vi "get Phasor Config.vi"(7 "phasorIndex":i32, 9 "pmuIndex":i32, 10 "pseudoPdcId":i32, 11 "phasorCfg":T1) -> (1 "function return":i32, 2 "name":string, 3 "phasorCfg out":T1)   [LabVIEW 2013, in "C37118-DLL.lvlib" / "StrongridDLL.lvlib"]
doc: "STRONGRIDIEEEC37118DLL_API int __cdecl getPhasorConfig(phasorConfig *phasorCfg, int32_t pseudoPdcId, int32_t pmuIndex, int32_t phasorIndex);"
uses:
  StrongridDLL.lvlib
  <vilib>/Utility/importsl/GetValueByPointer/datatype.ctl
  <vilib>/Utility/importsl/GetValueByPointer/GetValueByPointer.xnode
  StrongridDLL.dll
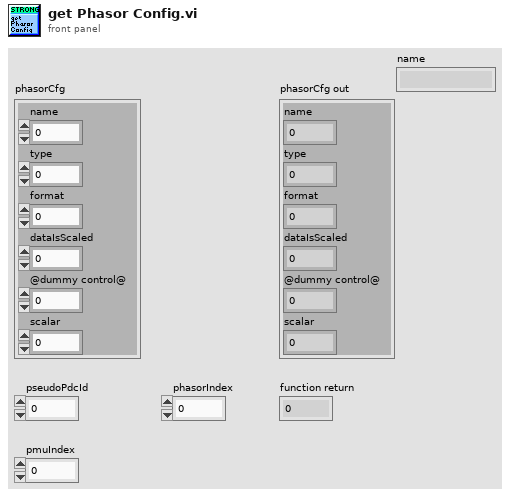
[diagram p1: front panel]
types:
  T1 = cluster{"name":u32, "type":u8, "format":u8, "dataIsScaled":u8, "@dummy control@":i8, "scalar":sgl}
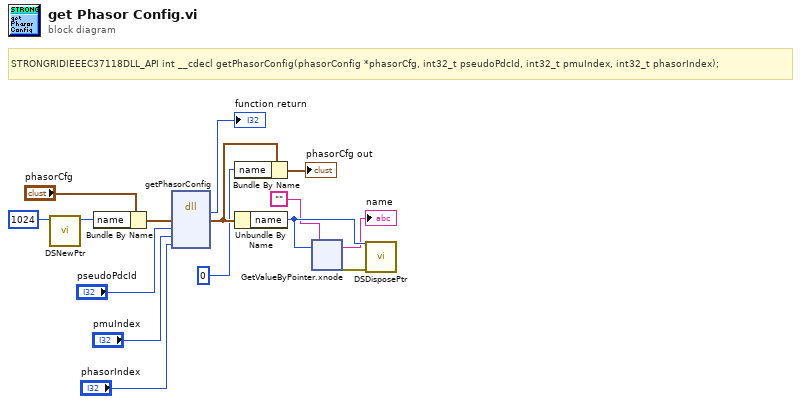
[diagram p0: block diagram]
diagram:
  # "STRONGRIDIEEEC37118DLL_API int __cdecl getPhasorConfig(phasorConfig *phasorCfg, int32_t pseudoPdcId, int32_t pmuIndex, int32_t phasorIndex);"
  n1 = call <vilib>:"DSNewPtr.vi"("Size"=u64 1024) -> ("Pointer"=w12:u64)  [unwired: 9 in, 1 out]
  n2 = Bundle By Name(cluster="phasorCfg", "name"=w12) -> (w11:T1)
  n3 = dll-call lib="C:/dev/statnett/S3DK-Startup/LabVIEW PRL Library LV2013/c37118-dll/labview/vi/Auto Generated/StrongridDLL.*" fn="getPhasorConfig"("phasorCfg"=w11, "pseudoPdcId"="pseudoPdcId", "pmuIndex"="pmuIndex", "phasorIndex"="phasorIndex") -> (→"function return":i32, "phasorCfg"=w6:T1)  [unwired: 6 in, 2 out]
  n4 = Bundle By Name(cluster=w6, "name"=u32 0) -> (→"phasorCfg out":T1)
  n5 = Unbundle By Name(w6) -> ("name"=w9:u32)
  n6 = xnode "GetValueByPointer.xnode"("Pointer"=w9, "InputType"="") -> ("Output"=→"name":string, "ErrorOut"=w10:errorcluster)  [unwired: 2 in]
  n7 = call <vilib>:"DSDisposePtr.vi"("error in (no error)"=w10, "Pointer"=w9) -> ()  [unwired: 9 in, 1 out]
